vi "SA40144E.20210819 1D + 2D vacuum.vi"() -> ()   [LabVIEW 2020]
uses:
  <vilib>/Analysis/baseanly.llb/Mean (DBL).vi
  <userlib>/_OpenG.lib/file/file.llb/Build Path - Traditional__ogtk.vi
  <userlib>/LevyLab/LV to ITX/Data/Data.lvclass
  <userlib>/LevyLab/XY Utilities/xy_utilities.lvlib
  <vilib>/Analysis/NI_AALBase.lvlib
panel:
  in  "Tab Control":enum32{"Page 1", "Page 2"}(tab)
  out "Temp vs t":T1(graph)
  out "G4T vs t  2D":T1(graph)
  out "G2T vs t 2D":T1(graph)
  out "G4T vs t":T1(graph)
  out "G2T vs t":T1(graph)
  out "Lifespan vs Temp (hrs)":cluster{i32[], dbl[]}[](graph)
  out "Linear Fit 2T":T1(graph)
  out "Linear Fit 4T":T1(graph)
  out "Linear Fit 2D 4T":T1(graph)
  out "Arrhenius 0 V before T change":T1(graph)
  out "Arrhenius -50 V inc":T1(graph)
  out "Arrhenius -100 V":T1(graph)
  out "Arrhenius -50 V dec":T1(graph)
  out "Arrhenius middle 0":T1(graph)
  out "Arrhenius 50 V dec":T1(graph)
  out "Arrhenius 100 V":T1(graph)
  out "Arrhenius  50 V inc":T1(graph)
  out "Arrhenius - 0 V after T change":T1(graph)
  in  "Temps to keep (Lifespan)":i32=26
  in  "Source Voltage":dbl=0.01
  in  "Init Temp":i32=275
  in  "Temp Step":i32=5
  in  "Final Temp":i32=315
  in  "Data Folder":path=path "G:/My Drive/ansom/Data/PPMS 2/SA40144E.20210819/00 - test"
  in  "Trimming":i32=400
  in  "Update":bool
  in  "OK":bool
  out "error out":errorcluster
  in  "error in (no error)":errorcluster
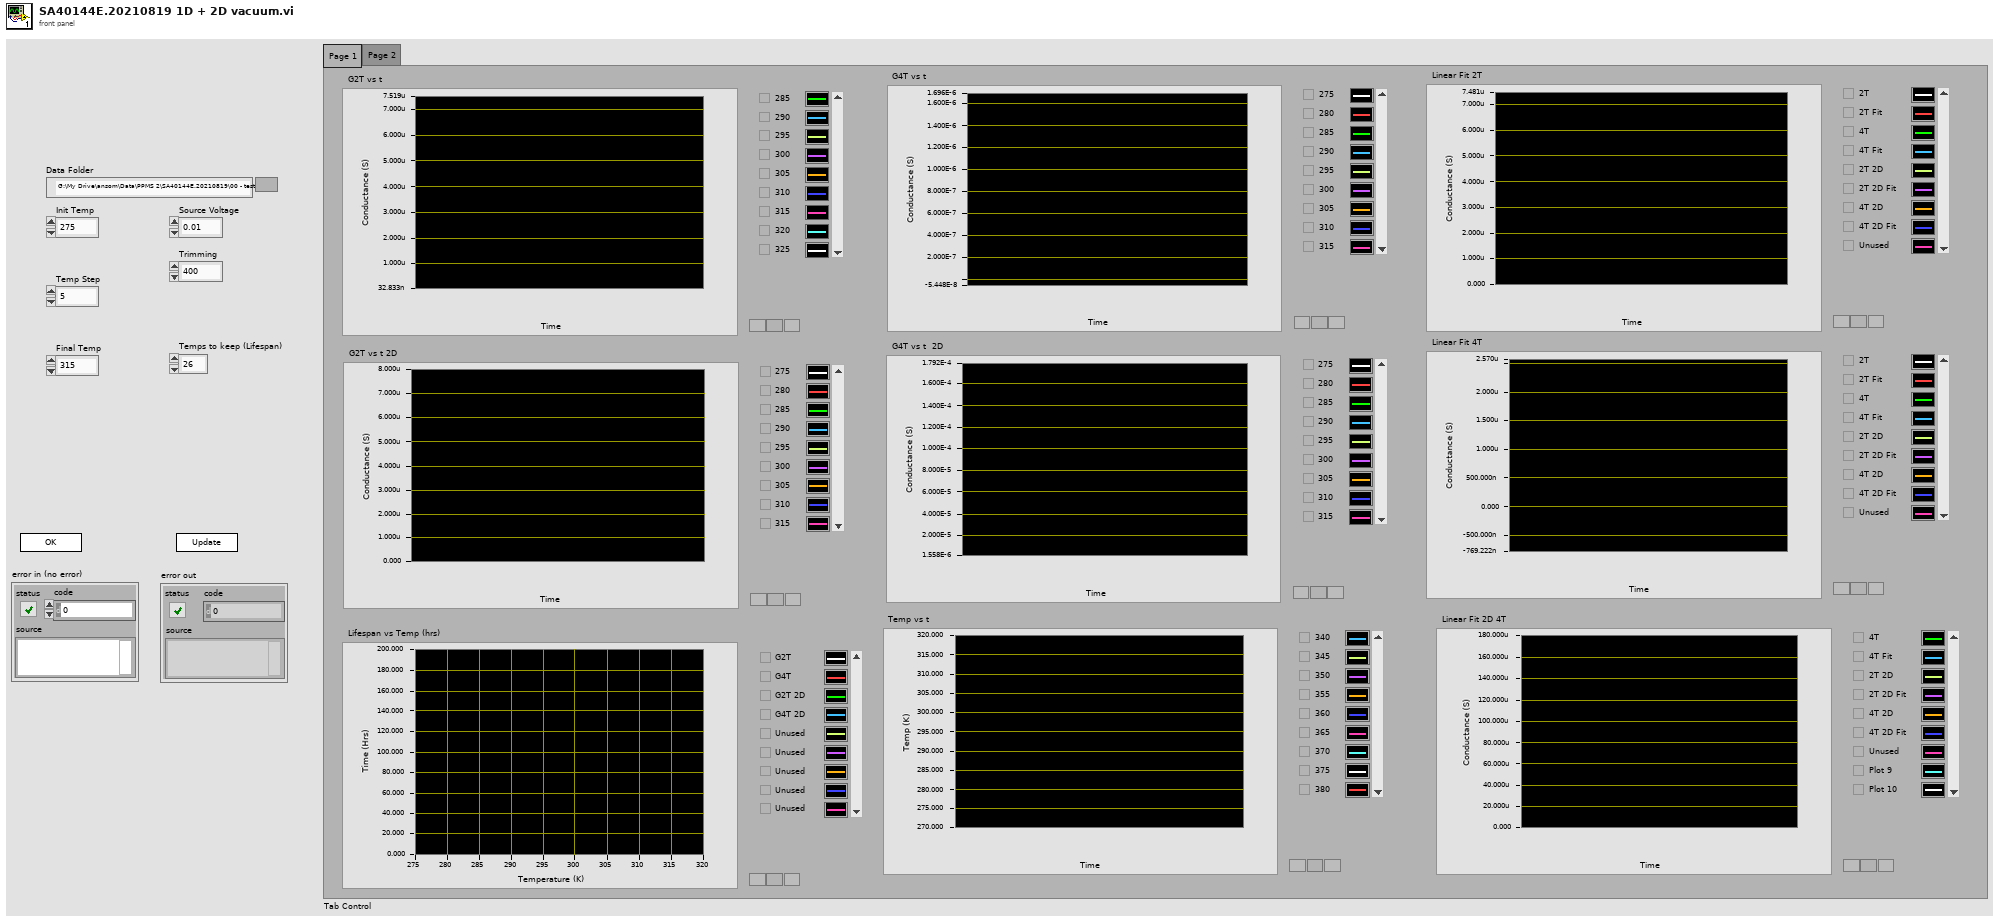
[diagram p1: front panel]
types:
  T1 = cluster{"Data":dbl[], "Best Exponential Fit":dbl[]}[]
  T2 = enum32{"Invalid", "Standard", "Closed", "Hidden", "Minimized", "Maximized"}
  T3 = enum32{"invalid app kind", "Development System", "Run Time System", "Student Edition", "Embedded LabVIEW", "Evaluation", "Custom"}
  T4 = cluster{"Core":cluster{"Current VI Reference":refnum<vi>, "Close Panel on Exit?":bool}, "G2T 1D":cluster{dbl[], dbl[]}[], "G4T 1D":cluster{dbl[], dbl[]}[], "G2T 2D":cluster{dbl[], dbl[]}[], "G4T 2D":cluster{dbl[], dbl[]}[], "Temp":cluster{dbl[], dbl[]}[], "Source Voltage":dbl, "Final Temp":i32, "Init Temp":i32, "Temp Step":i32, "Data Folder":path, "Trimming":i32}
  T5 = cluster{"Current VI Reference":refnum<vi>, "Close Panel on Exit?":bool}
  T6 = typedef "Data.lvclass/Dictionary--cluster.ctl" = cluster{"key":string, "value":variant}
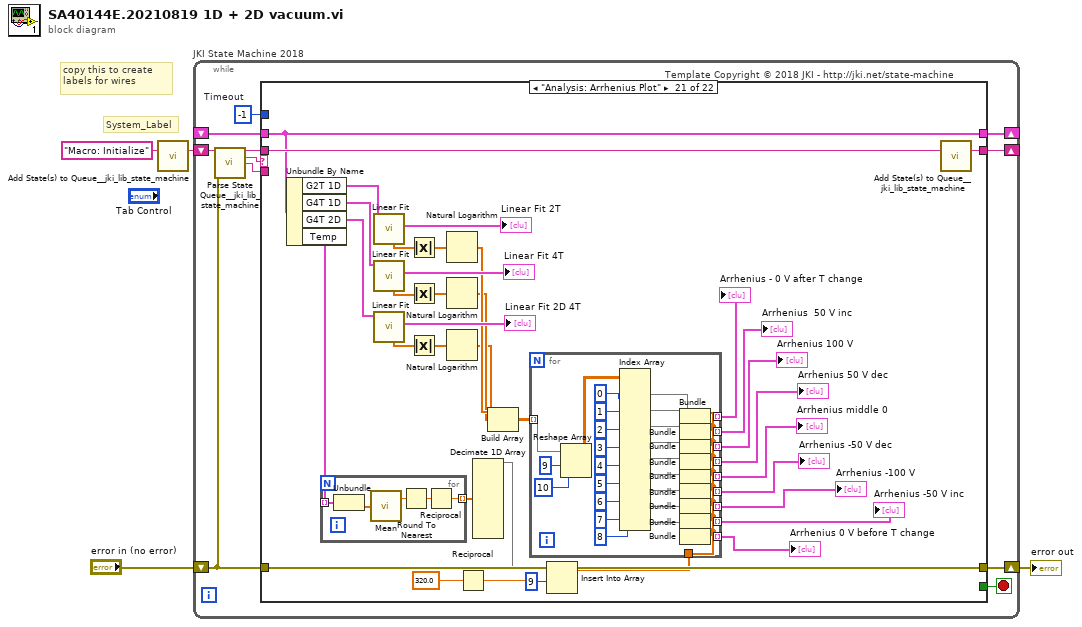
[diagram p0: block diagram]
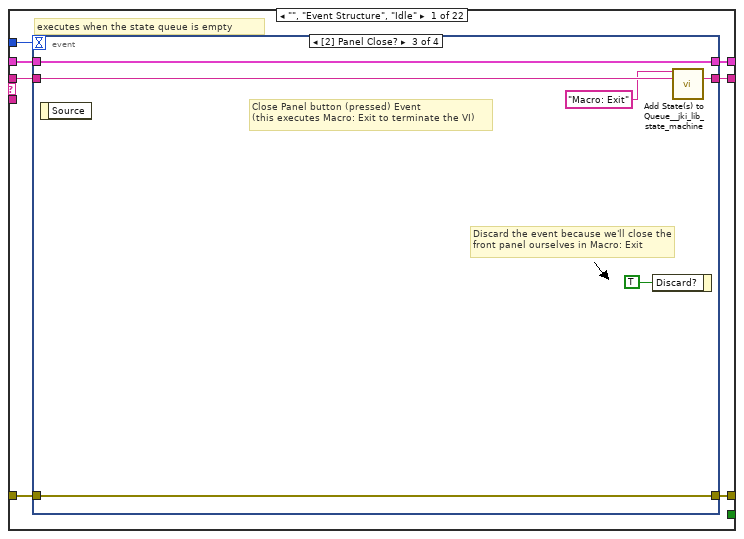
[diagram p2: hidden frame]
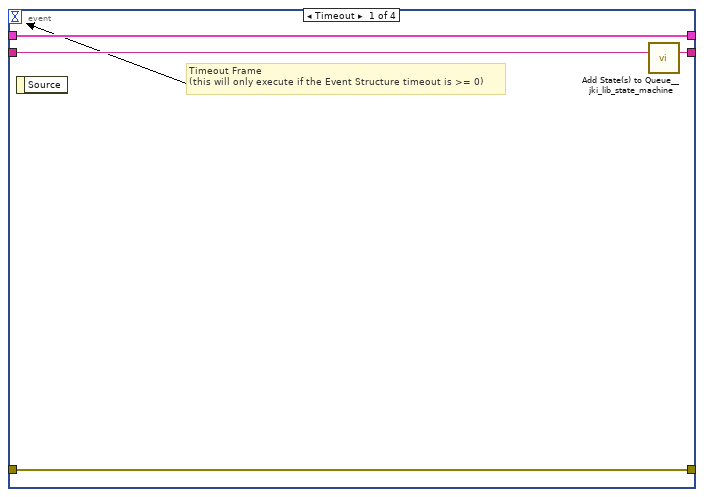
[diagram p3: hidden frame]
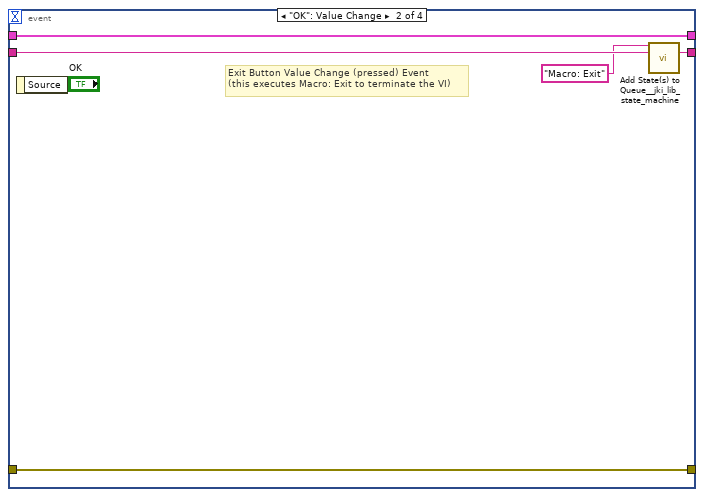
[diagram p4: hidden frame]
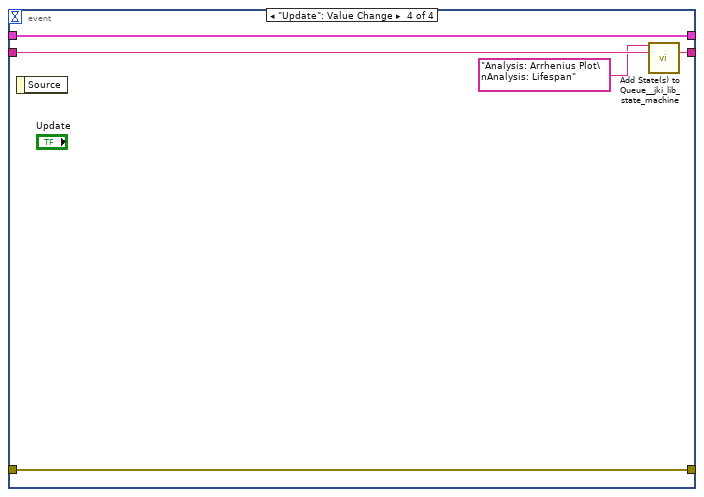
[diagram p5: hidden frame]
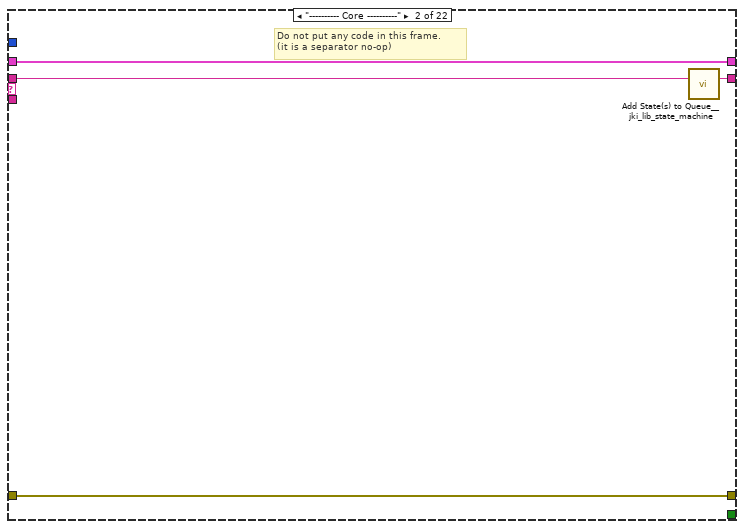
[diagram p6: hidden frame]
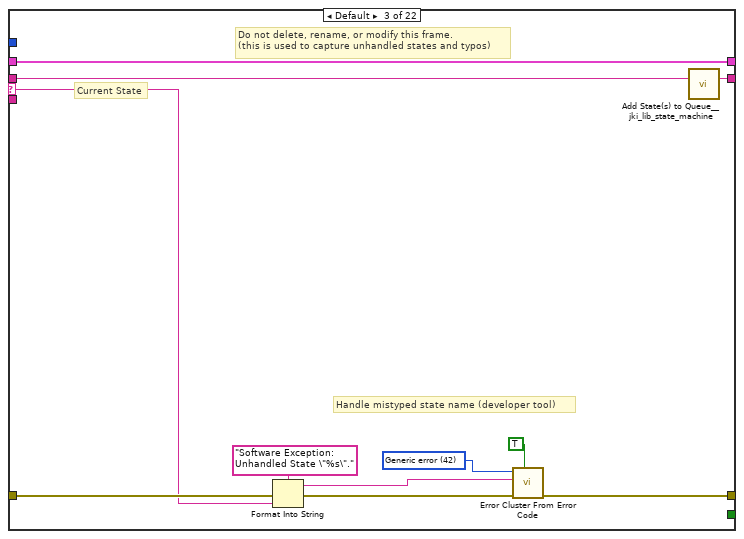
[diagram p7: hidden frame]
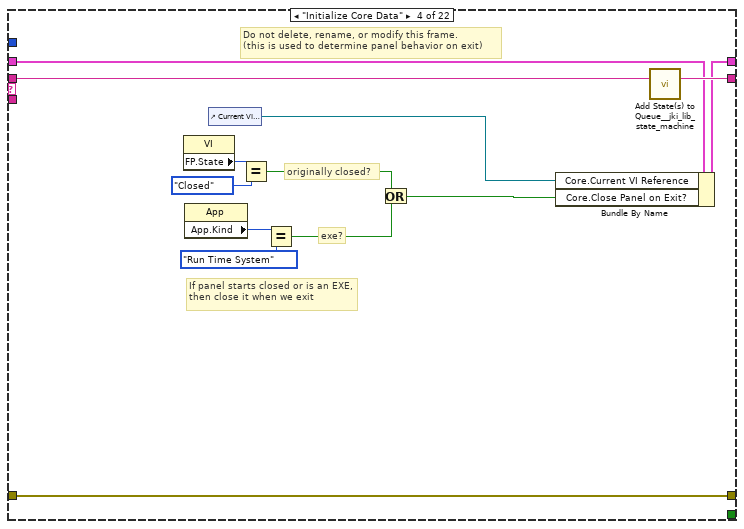
[diagram p8: hidden frame]
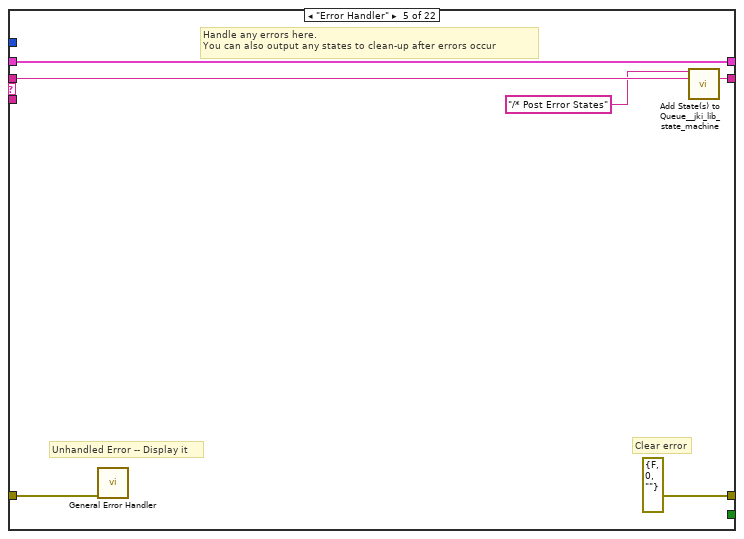
[diagram p9: hidden frame]
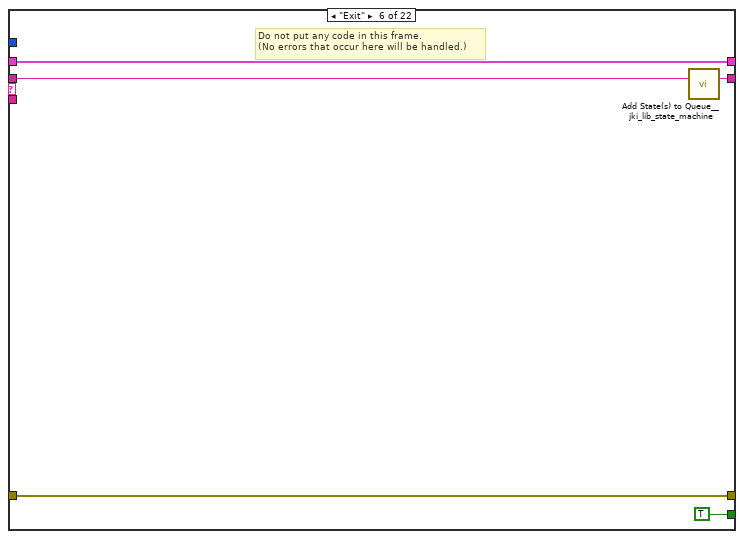
[diagram p10: hidden frame]
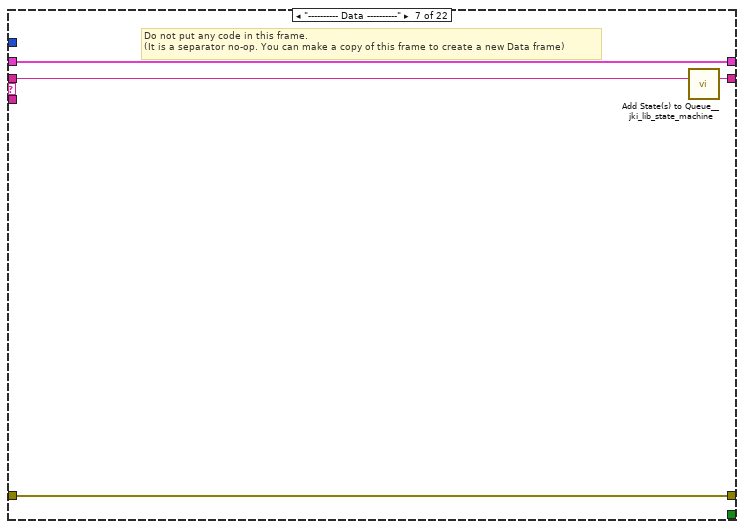
[diagram p11: hidden frame]
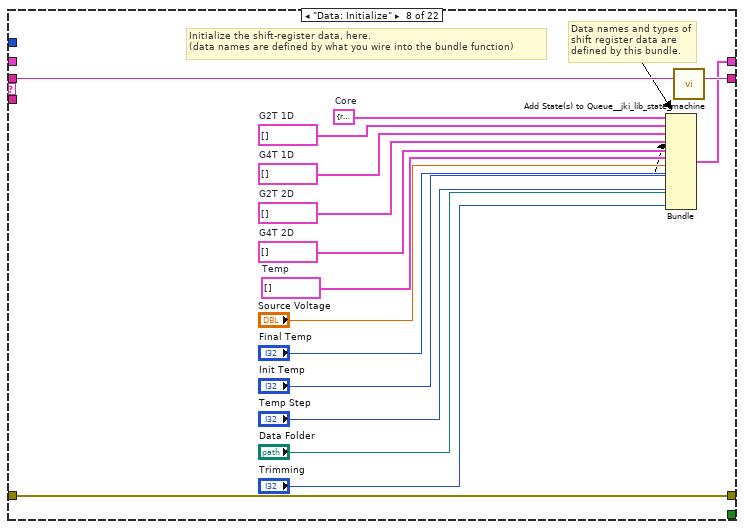
[diagram p12: hidden frame]
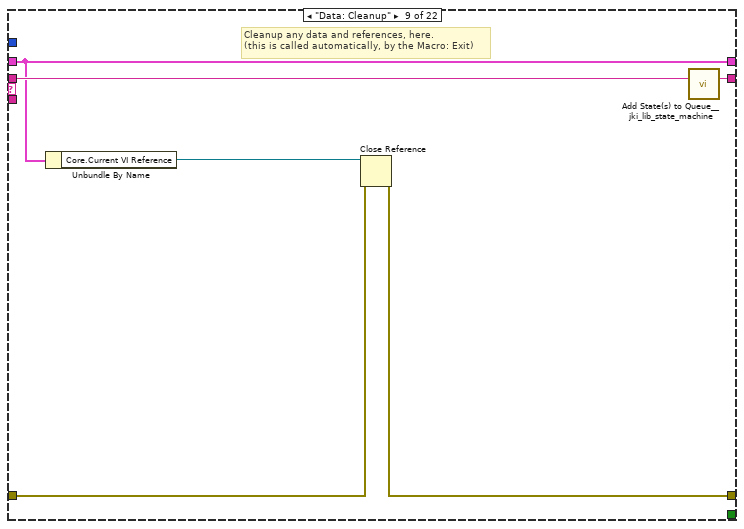
[diagram p13: hidden frame]
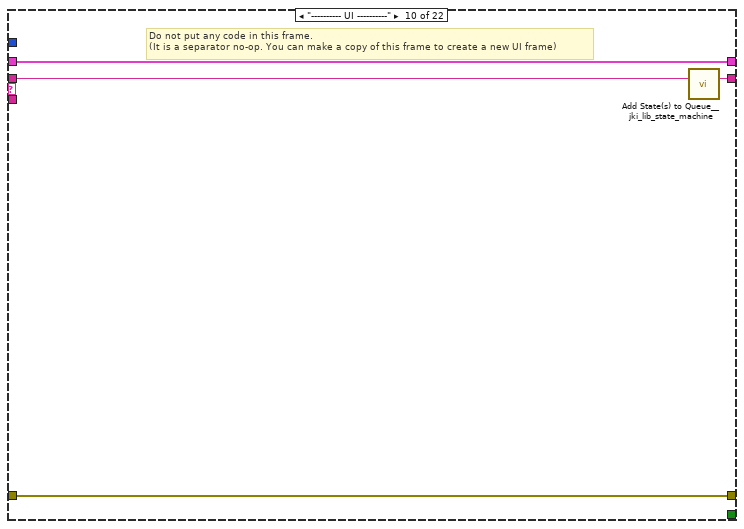
[diagram p14: hidden frame]
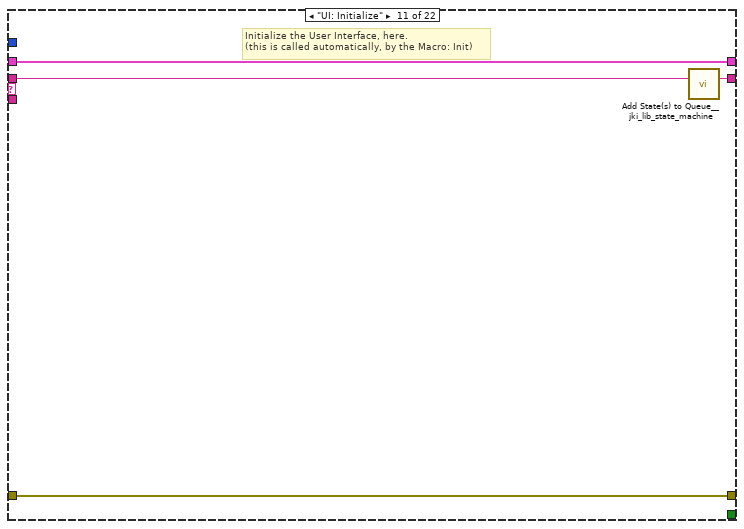
[diagram p15: hidden frame]
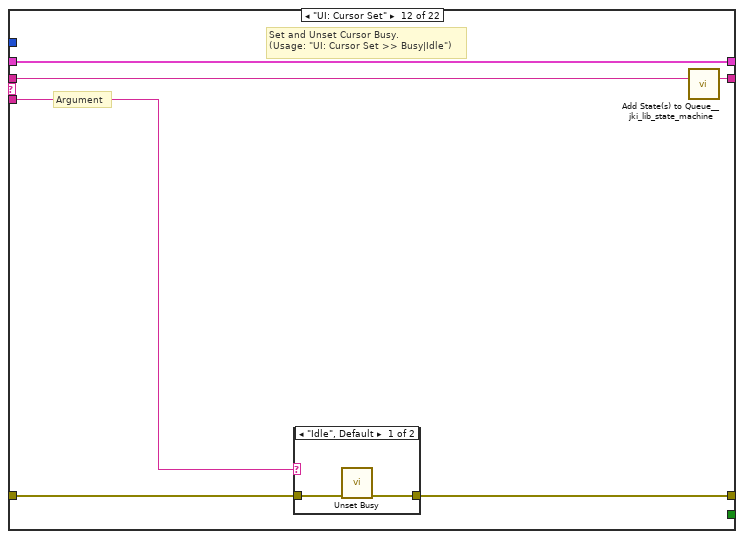
[diagram p16: hidden frame]
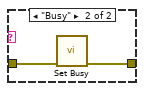
[diagram p17: hidden frame]
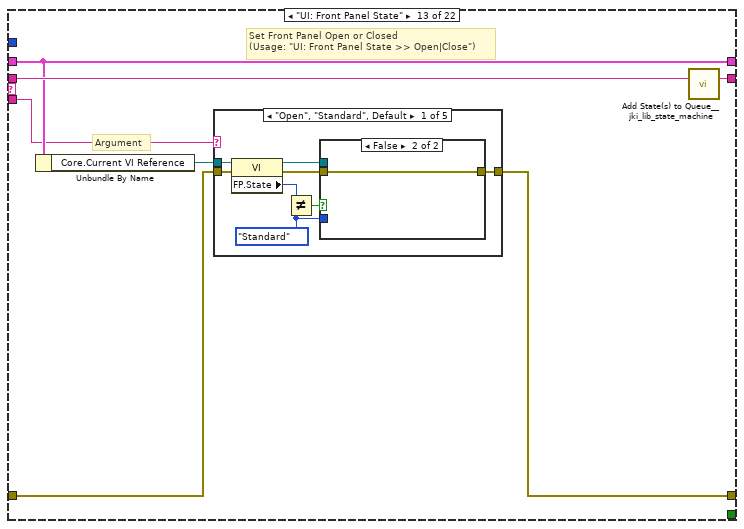
[diagram p18: hidden frame]
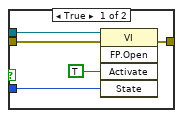
[diagram p19: hidden frame]
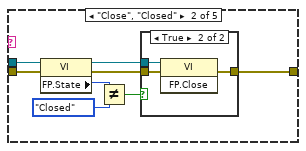
[diagram p20: hidden frame]
diagram:
  # "copy this to create labels for wires"
  # "System_Label"
  n1 = call <vilib>:"Add State(s) to Queue__jki_lib_state_machine.vi"("State(s) in (\"\")"="Macro: Initialize") -> ("States Out"=w4:string)  [unwired: 14 in]
  n2 = while "JKI State Machine 2018" {
    shift-right: [w8] -> _
    shift-left: _ -> [w7]
    shift-right: [w11] -> w1
    shift-left: "error in (no error)" -> [w5]
    shift-right: [w10] -> _
    shift-left: w4 -> [w12]
    stop <- w9 stop-if-true
    w6 = -1  # Timeout
    # "Template Copyright © 2018 JKI - http://jki.net/state-machine"
    n3 = call <vilib>:"Parse State Queue__jki_lib_state_machine.vi"("State Queue"=w12, "Error In (no error)"=w5) -> ("Remaining States"=w14:string, "Current State"=w15:string, "Arguments"=w13:string)  [unwired: 11 in]
    n4 = case shown="\"Analysis: Arrhenius Plot\"" w15 {
      selector: w15 -> [_ _ w47 _ _ _ _ _ _ _ _ _ _ _ _ _ _ _ _ _ _ _]
      tunnel: w14 -> [w22 w46 w51 w70 w76 w81 w85 w101 w107 w111 w115 w121 w132 w201 w206 w216 w220 w234 w274 w306 w342 w430]
      tunnel: w13 -> [_ _ _ _ _ _ _ _ _ _ _ w116 w126 _ _ _ _ _ _ _ _ _]
      tunnel: w7 -> [w20 w43 w49 w63 w73 w79 w82 _ w102 w108 w113 w119 w128 w198 w203 w213 w217 w230 w269 w303 w339 w410]
      tunnel: [w19 w44 w53 w67 errorcluster {"status"=FALSE, "code"=0, "source"=""} ("error out") w78 w83 w98 w103 w109 w112 w117 w129 w199 w204 w214 w218 w232 w272 w304 w340 w428] -> w11
      tunnel: w5 -> [w18 w44 w52 w67 w72 w78 w83 w98 w104 w109 w112 w118 w130 w199 w204 w214 w218 w232 w272 w304 w340 w428]
      tunnel: [w21 w45 w50 w69 w75 w80 w84 w100 w106 w110 w114 w120 w131 w200 w205 w215 w219 w233 w273 w305 w341 w429] -> w10
      tunnel: [_ _ _ _ _ TRUE _ _ _ _ _ _ _ _ _ _ _ _ _ _ _ _] -> w9
      tunnel: [w17 w43 w49 w68 w73 w79 w82 w99 w102 w108 w113 w119 w128 w198 w203 w213 w217 w231 w270 w303 w339 w410] -> w8
      tunnel: w6 -> [w16 _ _ _ _ _ _ _ _ _ _ _ _ _ _ _ _ _ _ _ _ _]
      frame "", "Event Structure", "Idle" {
        # "executes when the state queue is empty"
        n5 = event shown="[2] Panel Close?" {
          selector: _ -> [_ _ _ _]
          dyn-events: _ -> [_ _ _ _]
          timeout: w16 -> [_ _ _ _]
          tunnel: w22 -> [w26 w31 w37 w41]
          tunnel: [w25 w30 w36 w40] -> w21
          tunnel: w20 -> [w23 w28 w34 w42]
          tunnel: [w24 w29 w35 w38] -> w19
          tunnel: w18 -> [w24 w29 w35 w38]
          tunnel: [w23 w28 w34 w42] -> w17
          event Timeout {
            # "Timeout Frame\n(this will only execute if the Event Structure timeout is >= 0)"
            n6 = event-data() -> ()  [unwired: 1 in, 1 out]
            n7 = call <vilib>:"Add State(s) to Queue__jki_lib_state_machine.vi"("State(s) in (\"\")"=w26) -> ("States Out"=w25:string)  [unwired: 14 in]
          }
          event "OK": Value Change {
            # "Exit Button Value Change (pressed) Event\n(this executes Macro: Exit to terminate the VI)"
            n8 = event-data() -> ()  [unwired: 1 in, 1 out]
            n9 = call <vilib>:"Add State(s) to Queue__jki_lib_state_machine.vi"("State(s) in Front (\"\")"="Macro: Exit", "State(s) in (\"\")"=w31) -> ("States Out"=w30:string)  [unwired: 13 in]
          }
          event Panel Close? {
            # "Discard the event because we'll close the front panel ourselves in Macro: Exit"
            # "Close Panel button (pressed) Event\n(this executes Macro: Exit to terminate the VI)"
            n10 = event-data() -> ()  [unwired: 1 in, 1 out]
            n11 = event-data("Discard?"=TRUE) -> ()  [unwired: 1 in, 1 out]
            n12 = call <vilib>:"Add State(s) to Queue__jki_lib_state_machine.vi"("State(s) in Front (\"\")"="Macro: Exit", "State(s) in (\"\")"=w37) -> ("States Out"=w36:string)  [unwired: 13 in]
          }
          event "Update": Value Change {
            n13 = event-data() -> ()  [unwired: 1 in, 1 out]
            n14 = call <vilib>:"Add State(s) to Queue__jki_lib_state_machine.vi"("State(s) in Front (\"\")"="Analysis: Arrhenius Plot\nAnalysis: Lifespan" ("State(s) in Front (\"\")"), "State(s) in (\"\")"=w41) -> ("States Out"=w40:string)  [unwired: 13 in]
          }
        }
      }
      frame "---------- Core ----------" {
        # "Do not put any code in this frame.\n(it is a separator no-op)"
        n15 = call <vilib>:"Add State(s) to Queue__jki_lib_state_machine.vi"("State(s) in (\"\")"=w46) -> ("States Out"=w45:string)  [unwired: 14 in]
      }
      frame Default {
        w56 = 42 items=["No error", "Argument error", "Memory is full", "Out of zone", "End of file", "File already open", "Generic file I/O error", "File not found", "File permission error", "Disk is full", "Duplicate path", "Too many files open", "System feature not enabled", "Resource file not found", "Cannot add resource", "Resource not found", "Image not found", "Image memory error", "Pen does not exist", "Config type invalid", "Config token not found", "Config parse error", "Config memory error", "Bad external code format", "Bad external code offset", "External code not present", "Null window", "Destroy window error", "Null menu", "Print aborted", "Bad print record", "Print driver error", "Windows error during printing", "Memory error during printing", "Print dialog error", "Generic print error", "Invalid device refnum", "Device not found", "Device parameter error", "Device unit error", "Cannot open device", "Device call aborted", "Generic error", "Cancelled by user", "Object ID too low", "Object ID too high", "Object not in heap", "Unknown heap", "Unknown object (invalid DefProc)", "Unknown object (DefProc not in table)", "Message out of range", "Invalid (null) method", "Unknown message", "Manager call not supported", "Bad address", "Network operation in progress", "Network operation timed out", "Connection is busy", "Network attribute not supported", "Network error", "Address in use", "System out of memory", "Connection aborted", "Connection refused", "Not connected", "Already connected", "Connection closed", "Initialization error (interapplication manager)", "Bad occurrence", "Wait on unbound occurrence handler", "Occurrence queue overflow", "Datalog type conflict", "Unused", "Unrecognized type (interapplication manager)", "Memory corrupt", "Failed to make temporary DLL", "Old CIN version", "Drag socket not found", "Failed to load drop-object", "Failed to register OLE object", "Failed to release OLE object", "Format specifier type mismatch", "Unknown format specifier", "Too few format specifiers", "Too many format specifiers", "Scan failed", "Newer CIN version", "Error converting to variant", "Runtime menu error", "Password tampered", "Variant attribute not found", "Incompatible variant data type", "Event data is not available", "Event Store is not present", "Occurrence is not found", "Event Queue is not created", "Event info is not available", "Refnum passed is NULL", "Error retrieving Class GUID", "Error retrieving CoClass GUID", "Error retrieving TypeLib GUID.", "Bad built application magic bytes.", "Specific driver is different from the specific driver associated with the Logical Name.", "There is no session opened to the class driver.", "Max Error", "MAX - Error with config objects", "MAX - Error loading configuration", "MAX - Group not supported"]
        # "Current State"
        # "Do not delete, rename, or modify this frame.\n(this is used to capture unhandled states and typos)"
        # "Handle mistyped state name (developer tool)"
        n16 = Format Into String(format string="Software Exception: Unhandled State \"%s\"." ("message"), error in=w52, w47) -> (resulting string=w55:string, error out=w54:errorcluster)  [unwired: 1 in]
        n17 = call <vilib>:"Error Cluster From Error Code.vi"("show call chain? (False)"=TRUE, "error in (no error)"=w54, "error message (\"\")"=w55, "error code (0)"=w56) -> ("error out"=w53:errorcluster)  [unwired: 5 in]
        n18 = call <vilib>:"Add State(s) to Queue__jki_lib_state_machine.vi"("State(s) in (\"\")"=w51) -> ("States Out"=w50:string)  [unwired: 14 in]
      }
      frame "Initialize Core Data" {
        # "Do not delete, rename, or modify this frame.\n(this is used to determine panel behavior on exit)"
        # "originally closed?"
        # "exe?"
        # "If panel starts closed or is an EXE, then close it when we exit"
        n19 = property class="VI"() -> ("FP.State"=w60:T2)  [unwired: 2 in, 2 out]
        n20 = property class="App"() -> ("App.Kind"=w66:T3)  [unwired: 2 in, 2 out]
        n21 = control-ref of="Current VI Reference"() -> (w61:refnum<vi>)
        n22 = Equal?(x=w60, y=T2."Closed" ("Front Panel Window:State")) -> (x = y?=w58:bool)
        n23 = Equal?(x=w66, y=T3."Run Time System" ("Application:Kind")) -> (x = y?=w64:bool)
        n24 = Or(x=w58, y=w64) -> (x .or. y?=w62:bool)
        n25 = Bundle By Name(cluster=w63, "Core.Current VI Reference"=w61, "Core.Close Panel on Exit?"=w62) -> (w68:T4)
        n26 = call <vilib>:"Add State(s) to Queue__jki_lib_state_machine.vi"("State(s) in (\"\")"=w70) -> ("States Out"=w69:string)  [unwired: 14 in]
      }
      frame "Error Handler" {
        # "Unhandled Error -- Display it"
        # "Handle any errors here.\nYou can also output any states to clean-up after errors occur"
        # "Clear error"
        n27 = call <vilib>:"General Error Handler.vi"("error in (no error)"=w72) -> ()  [unwired: 10 in, 5 out]
        n28 = call <vilib>:"Add State(s) to Queue__jki_lib_state_machine.vi"("State(s) in Front (\"\")"="/* Post Error States", "State(s) in (\"\")"=w76) -> ("States Out"=w75:string)  [unwired: 13 in]
      }
      frame "Exit" {
        # "Do not put any code in this frame.\n(No errors that occur here will be handled.)"
        n29 = call <vilib>:"Add State(s) to Queue__jki_lib_state_machine.vi"("State(s) in (\"\")"=w81) -> ("States Out"=w80:string)  [unwired: 14 in]
      }
      frame "---------- Data ----------" {
        # "Do not put any code in this frame.\n(It is a separator no-op. You can make a copy of this frame to create a new Data frame)"
        n30 = call <vilib>:"Add State(s) to Queue__jki_lib_state_machine.vi"("State(s) in (\"\")"=w85) -> ("States Out"=w84:string)  [unwired: 14 in]
      }
      frame "Data: Initialize" {
        w86 = cluster{dbl[], dbl[]}[] []  # Temp
        w95 = cluster{dbl[], dbl[]}[] []  # G4T 2D
        w94 = cluster{dbl[], dbl[]}[] []  # G2T 2D
        w93 = cluster{dbl[], dbl[]}[] []  # G4T 1D
        w92 = cluster{dbl[], dbl[]}[] []  # G2T 1D
        w97 = T5 {"Current VI Reference"=refnum, "Close Panel on Exit?"=FALSE}  # Core
        # "Data names and types of shift register data are defined by this bundle."
        # "Initialize the shift-register data, here.\n(data names are defined by what you wire into the bundle function)"
        n31 = Bundle("Core"=w97, "G2T 1D"=w92, "G4T 1D"=w93, "G2T 2D"=w94, "G4T 2D"=w95, "Temp"=w86, "Source Voltage"="Source Voltage", "Final Temp"="Final Temp", "Init Temp"="Init Temp", "Temp Step"="Temp Step", "Data Folder"="Data Folder", "Trimming"="Trimming") -> (w99:T4)  [unwired: 1 in]
        n32 = call <vilib>:"Add State(s) to Queue__jki_lib_state_machine.vi"("State(s) in (\"\")"=w101) -> ("States Out"=w100:string)  [unwired: 14 in]
      }
      frame "Data: Cleanup" {
        # "Cleanup any data and references, here.\n(this is called automatically, by the Macro: Exit)"
        n33 = Unbundle By Name(w102) -> ("Core.Current VI Reference"=w105:refnum<vi>)
        n34 = Close Reference(reference=w105, error in (no error)=w104) -> (error out=w103:errorcluster)
        n35 = call <vilib>:"Add State(s) to Queue__jki_lib_state_machine.vi"("State(s) in (\"\")"=w107) -> ("States Out"=w106:string)  [unwired: 14 in]
      }
      frame "---------- UI ----------" {
        # "Do not put any code in this frame.\n(It is a separator no-op. You can make a copy of this frame to create a new UI frame)"
        n36 = call <vilib>:"Add State(s) to Queue__jki_lib_state_machine.vi"("State(s) in (\"\")"=w111) -> ("States Out"=w110:string)  [unwired: 14 in]
      }
      frame "UI: Initialize" {
        # "Initialize the User Interface, here.\n(this is called automatically, by the Macro: Init)"
        n37 = call <vilib>:"Add State(s) to Queue__jki_lib_state_machine.vi"("State(s) in (\"\")"=w115) -> ("States Out"=w114:string)  [unwired: 14 in]
      }
      frame "UI: Cursor Set" {
        # "Argument"
        # "Set and Unset Cursor Busy.\n(Usage: \"UI: Cursor Set >> Busy|Idle\")"
        n38 = case shown="\"Idle\", Default" w116 {
          tunnel: w118 -> [w123 w125]
          tunnel: [w122 w124] -> w117
          frame "Idle", Default {
            n39 = call <vilib>:"Unset Busy.vi"("error in (no error)"=w123) -> ("error out"=w122:errorcluster)  [unwired: 10 in]
          }
          frame "Busy" {
            n40 = call <vilib>:"Set Busy.vi"("error in (no error)"=w125) -> ("error out"=w124:errorcluster)  [unwired: 9 in, 1 out]
          }
        }
        n41 = call <vilib>:"Add State(s) to Queue__jki_lib_state_machine.vi"("State(s) in (\"\")"=w121) -> ("States Out"=w120:string)  [unwired: 14 in]
      }
      frame "UI: Front Panel State" {
        # "Argument"
        # "Set Front Panel Open or Closed\n(Usage: \"UI: Front Panel State >> Open|Close\")"
        n42 = Unbundle By Name(w128) -> ("Core.Current VI Reference"=w127:refnum<vi>)
        n43 = case shown="\"Open\", \"Standard\", Default" w126 {
          tunnel: w130 -> [w138 w153 w164 w177 w190]
          tunnel: [w140 w154 w166 w179 w192] -> w129
          tunnel: w127 -> [w139 w151 w165 w178 w191]
          frame "Open", "Standard", Default {
            w133 = T2."Standard" ("State")
            n44 = property class="VI"(reference=w139, error in=w138) -> (reference out=w136:refnum<vi>, error out=w137:errorcluster, "FP.State"=w135:T2)
            n45 = Not Equal?(x=w135, y=w133) -> (x != y?=w134:bool)
            n46 = case shown="False" w134 {
              tunnel: [w144 w146] -> w140
              tunnel: w137 -> [w143 w146]
              tunnel: w136 -> [w142 _]
              tunnel: w133 -> [w141 _]
              frame True {
                n47 = invoke class="VI" method="FP.Open"(reference=w142, error in=w143, "Activate"=TRUE, "State"=w141) -> (error out=w144:errorcluster)  [unwired: 1 in, 4 out]
              }
              frame False {
              }
            }
          }
          frame "Close", "Closed" {
            n48 = property class="VI"(reference=w151, error in=w153) -> (reference out=w150:refnum<vi>, error out=w152:errorcluster, "FP.State"=w148:T2)
            n49 = Not Equal?(x=w148, y=T2."Closed" ("Front Panel Window:State")) -> (x != y?=w147:bool)
            n50 = case shown="True" w147 {
              tunnel: [w155 w158] -> w154
              tunnel: w152 -> [w155 w157]
              tunnel: w150 -> [_ w156]
              frame False {
              }
              frame True {
                n51 = invoke class="VI" method="FP.Close"(reference=w156, error in=w157) -> (error out=w158:errorcluster)  [unwired: 1 in, 2 out]
              }
            }
          }
          frame "Hidden", "Hide" {
            w159 = T2."Hidden" ("State")
            n52 = property class="VI"(reference=w165, error in=w164) -> (reference out=w162:refnum<vi>, error out=w163:errorcluster, "FP.State"=w161:T2)
            n53 = Not Equal?(x=w161, y=w159) -> (x != y?=w160:bool)
            n54 = case shown="True" w160 {
              tunnel: [w170 w171] -> w166
              tunnel: w163 -> [w169 w171]
              tunnel: w162 -> [w168 _]
              tunnel: w159 -> [w167 _]
              frame True {
                n55 = invoke class="VI" method="FP.Open"(reference=w168, error in=w169, "State"=w167) -> (error out=w170:errorcluster)  [unwired: 2 in, 4 out]
              }
              frame False {
              }
            }
          }
          frame "Minimize", "Minimized" {
            w172 = T2."Minimized" ("State")
            n56 = property class="VI"(reference=w178, error in=w177) -> (reference out=w175:refnum<vi>, error out=w176:errorcluster, "FP.State"=w174:T2)
            n57 = Not Equal?(x=w174, y=w172) -> (x != y?=w173:bool)
            n58 = case shown="True" w173 {
              tunnel: [w183 w184] -> w179
              tunnel: w176 -> [w182 w184]
              tunnel: w175 -> [w181 _]
              tunnel: w172 -> [w180 _]
              frame True {
                n59 = invoke class="VI" method="FP.Open"(reference=w181, error in=w182, "State"=w180) -> (error out=w183:errorcluster)  [unwired: 2 in, 4 out]
              }
              frame False {
              }
            }
          }
          frame "Maximize", "Maximized" {
            w185 = T2."Maximized" ("State")
            n60 = property class="VI"(reference=w191, error in=w190) -> (reference out=w188:refnum<vi>, error out=w189:errorcluster, "FP.State"=w187:T2)
            n61 = Not Equal?(x=w187, y=w185) -> (x != y?=w186:bool)
            n62 = case shown="True" w186 {
              tunnel: [w196 w197] -> w192
              tunnel: w189 -> [w195 w197]
              tunnel: w188 -> [w194 _]
              tunnel: w185 -> [w193 _]
              frame True {
                n63 = invoke class="VI" method="FP.Open"(reference=w194, error in=w195, "State"=w193) -> (error out=w196:errorcluster)  [unwired: 2 in, 4 out]
              }
              frame False {
              }
            }
          }
        }
        n64 = call <vilib>:"Add State(s) to Queue__jki_lib_state_machine.vi"("State(s) in (\"\")"=w132) -> ("States Out"=w131:string)  [unwired: 14 in]
      }
      frame "---------- Macro ----------" {
        # "Do not put any code in this frame.\n(It is a separator no-op. You can make a copy of this frame to create a new Macro frame)"
        n65 = call <vilib>:"Add State(s) to Queue__jki_lib_state_machine.vi"("State(s) in (\"\")"=w201) -> ("States Out"=w200:string)  [unwired: 14 in]
      }
      frame "Macro: Initialize" {
        # "Initialization Macro\n(This is called once, when the VI starts)"
        n66 = call <vilib>:"Add State(s) to Queue__jki_lib_state_machine.vi"("State(s) in Front (\"\")"="Data: Initialize\nInitialize Core Data\nUI: Initialize\nUI: Front Panel State >> Open\nAnalysis: Load 1D\nAnalysis: Load 2D\nAnalysis: Plot G vs t\nAnalysis: Arrhenius Plot\n# Analysis: Lifespan", "State(s) in (\"\")"=w206) -> ("States Out"=w205:string)  [unwired: 13 in]
      }
      frame "Macro: Exit" {
        # "Exit Macro\n(This is called once, when the VI exits)"
        n67 = Unbundle By Name(w213) -> ("Core.Close Panel on Exit?"=w212:bool)
        n68 = Select(t="UI: Front Panel State >> Close", s=w212, f="") -> (s? t:f=w209:string)
        n69 = call <vilib>:"Add State(s) to Queue__jki_lib_state_machine.vi"("State(s) in (\"\")"=w209, "State(s) at Back (\"\")"="Data: Cleanup\nExit") -> ("States Out"=w207:string)  [unwired: 13 in]
        n70 = call <vilib>:"Add State(s) to Queue__jki_lib_state_machine.vi"("State(s) in Front (\"\")"=w207, "State(s) in (\"\")"=w216) -> ("States Out"=w215:string)  [unwired: 13 in]
      }
      frame "---------- Analysis ----------" {
        # "Template Separator\n(You can make a copy of, or modify, this frame)"
        n71 = call <vilib>:"Add State(s) to Queue__jki_lib_state_machine.vi"("State(s) in (\"\")"=w220) -> ("States Out"=w219:string)  [unwired: 14 in]
      }
      frame "Analysis: Load 1D" {
        # "G2T = X3/V_s\nG4T = X3/(X5-X4)"
        n72 = Unbundle By Name(w230) -> ("Source Voltage"=w229:dbl, "Trimming"=w225:i32, "Data Folder"=w226:path)
        n73 = List Folder(path=w226, pattern="*.dat") -> (path out=w224:path, filenames=w223:string[])  [unwired: 2 in, 2 out]
        n74 = for {
          tunnel: w229 -> [w240]
          tunnel: [w261] -> w228 mode=indexing
          tunnel: [w260] -> w222 mode=indexing
          tunnel: w225 -> [w246]
          tunnel: [w258] -> w227 mode=indexing
          tunnel: w224 -> [w245]
          tunnel: w223 -> [w244] mode=indexing
          n75 = call-poly <userlib>:"Build Path__ogtk.vi"("name or relative path"=w244, "base path"=w245) -> ("appended path"=w243:path)
          n76 = call <userlib>:"Data Read.vi"("path"=w243) -> ("Data (Dictionary)"=w257:T6[])  [unwired: 7 in, 3 out]
          n77 = call "Read Dictionary.vi"("Numeric"=0, "Dictionary In"=w257) -> ("data"=w253:dbl[])
          n78 = call "Read Dictionary.vi"("Numeric"=5, "Dictionary In"=w257) -> ("data"=w247:dbl[])
          n79 = call "Read Dictionary.vi"("Numeric"=7 ("index"), "Dictionary In"=w257) -> ("data"=w248:dbl[])
          n80 = call "Read Dictionary.vi"("Numeric"=6, "Dictionary In"=w257) -> ("data"=w252:dbl[])
          n81 = call "Read Dictionary.vi"("Numeric"=1, "Dictionary In"=w257) -> ("data"=w251:dbl[])
          n82 = Array Subset(array=w253, index=w246) -> (w242:dbl[])  [unwired: 1 in]
          n83 = Array Subset(array=w247, index=w246) -> (w237:dbl[])  [unwired: 1 in]
          n84 = Array Subset(array=w248, index=w246) -> (w239:dbl[])  [unwired: 1 in]
          n85 = Array Subset(array=w252, index=w246) -> (w238:dbl[])  [unwired: 1 in]
          n86 = Subtract(x=w239, y=w238) -> (x-y=w236:dbl[])
          n87 = Divide(x=w237, y=w240) -> (x/y=w241:dbl[])
          n88 = Divide(x=w237, y=w236) -> (x/y=w235:dbl[])
          n89 = Array Subset(array=w251) -> (w259:dbl[])  [unwired: 2 in]
          n90 = Bundle(w242, w241) -> (w261:cluster{dbl[], dbl[]})  [unwired: 1 in]
          n91 = Bundle(w242, w259) -> (w258:cluster{dbl[], dbl[]})  [unwired: 1 in]
          n92 = Bundle(w242, w235) -> (w260:cluster{dbl[], dbl[]})  [unwired: 1 in]
        }
        n93 = call <vilib>:"Add State(s) to Queue__jki_lib_state_machine.vi"("State(s) in (\"\")"=w234) -> ("States Out"=w233:string)  [unwired: 14 in]
        n94 = Bundle By Name(cluster=w230, "G2T 1D"=w228, "G4T 1D"=w222, "Temp"=w227) -> (w231:T4)
      }
      frame "Analysis: Load 2D" {
        # "G2T = X3/V_s\nG4T = X3/(X8-X1)"
        n95 = Unbundle By Name(w269) -> ("Source Voltage"=w271:dbl, "Trimming"=w268:i32, "Data Folder"=w267:path)
        n96 = List Folder(path=w267, pattern="*.dat") -> (path out=w266:path, filenames=w265:string[])  [unwired: 2 in, 2 out]
        n97 = for {
          tunnel: w271 -> [w279]
          tunnel: [w296] -> w264 mode=indexing
          tunnel: [w295] -> w263 mode=indexing
          tunnel: w268 -> [w294]
          tunnel: w266 -> [w283]
          tunnel: w265 -> [w282] mode=indexing
          n98 = call-poly <userlib>:"Build Path__ogtk.vi"("name or relative path"=w282, "base path"=w283) -> ("appended path"=w297:path)
          n99 = call <userlib>:"Data Read.vi"("path"=w297) -> ("Data (Dictionary)"=w292:T6[])  [unwired: 7 in, 3 out]
          n100 = call "Read Dictionary.vi"("Numeric"=0, "Dictionary In"=w292) -> ("data"=w291:dbl[])
          n101 = call "Read Dictionary.vi"("Numeric"=5, "Dictionary In"=w292) -> ("data"=w288:dbl[])
          n102 = call "Read Dictionary.vi"("Numeric"=3 ("index"), "Dictionary In"=w292) -> ("data"=w289:dbl[])
          n103 = call "Read Dictionary.vi"("Numeric"=4, "Dictionary In"=w292) -> ("data"=w290:dbl[])
          n104 = Array Subset(array=w291, index=w294) -> (w293:dbl[])  [unwired: 1 in]
          n105 = Array Subset(array=w288, index=w294) -> (w280:dbl[])  [unwired: 1 in]
          n106 = Array Subset(array=w289, index=w294) -> (w278:dbl[])  [unwired: 1 in]
          n107 = Array Subset(array=w290, index=w294) -> (w277:dbl[])  [unwired: 1 in]
          n108 = Subtract(x=w278, y=w277) -> (x-y=w281:dbl[])
          n109 = Divide(x=w280, y=w279) -> (x/y=w275:dbl[])
          n110 = Divide(x=w280, y=w281) -> (x/y=w276:dbl[])
          n111 = Bundle(w293, w275) -> (w296:cluster{dbl[], dbl[]})  [unwired: 1 in]
          n112 = Bundle(w293, w276) -> (w295:cluster{dbl[], dbl[]})  [unwired: 1 in]
        }
        n113 = call <vilib>:"Add State(s) to Queue__jki_lib_state_machine.vi"("State(s) in (\"\")"=w274) -> ("States Out"=w273:string)  [unwired: 14 in]
        n114 = Bundle By Name(cluster=w269, "G2T 2D"=w264, "G4T 2D"=w263) -> (w270:T4)
      }
      frame "Analysis: Plot G vs t" {
        n115 = Unbundle By Name(w303) -> ("G2T 1D"=→"G2T vs t":cluster{dbl[], dbl[]}[], "G4T 1D"=→"G4T vs t":cluster{dbl[], dbl[]}[], "G2T 2D"=→"G2T vs t 2D":cluster{dbl[], dbl[]}[], "G4T 2D"=→"G4T vs t  2D":cluster{dbl[], dbl[]}[], "Temp"=→"Temp vs t":cluster{dbl[], dbl[]}[])
        n116 = call <vilib>:"Add State(s) to Queue__jki_lib_state_machine.vi"("State(s) in (\"\")"=w306) -> ("States Out"=w305:string)  [unwired: 14 in]
      }
      frame "Analysis: Arrhenius Plot" {
        n117 = Unbundle By Name(w339) -> ("G2T 1D"=w336:cluster{dbl[], dbl[]}[], "G4T 1D"=w335:cluster{dbl[], dbl[]}[], "G4T 2D"=w338:cluster{dbl[], dbl[]}[], "Temp"=w329:cluster{dbl[], dbl[]}[])
        n118 = for {
          tunnel: w329 -> [w379] mode=indexing
          tunnel: [w377] -> w321 mode=indexing
          n119 = Unbundle(w379) -> (w376:dbl[])  [unwired: 1 out]
          n120 = call-poly <vilib>:"Mean.vi"("X"=w376) -> ("mean"=w375:dbl)  [unwired: 1 out]
          n121 = Round To Nearest(number=w375) -> (nearest integer value=w378:dbl)
          n122 = Reciprocal(x=w378) -> (1/x=w377:dbl)
        }
        n123 = call-poly <userlib>:"Linear Fit.vi"("XY-data"=w336) -> ("Best Fits"=→"Linear Fit 2T":cluster{"X-array":dbl[], "Y-array":dbl[]}[], "slopes"=w333:dbl[])  [unwired: 4 in, 5 out]
        n124 = call-poly <userlib>:"Linear Fit.vi"("XY-data"=w335) -> ("Best Fits"=→"Linear Fit 4T":cluster{"X-array":dbl[], "Y-array":dbl[]}[], "slopes"=w334:dbl[])  [unwired: 4 in, 5 out]
        n125 = call-poly <userlib>:"Linear Fit.vi"("XY-data"=w338) -> ("Best Fits"=→"Linear Fit 2D 4T":cluster{"X-array":dbl[], "Y-array":dbl[]}[], "slopes"=w337:dbl[])  [unwired: 4 in, 5 out]
        n126 = Absolute Value(x=w333) -> (abs(x)=w328:dbl[])
        n127 = Absolute Value(x=w334) -> (abs(x)=w327:dbl[])
        n128 = Absolute Value(x=w337) -> (abs(x)=w326:dbl[])
        n129 = Natural Logarithm(1:w328) -> (0:w324:dbl[])
        n130 = Natural Logarithm(1:w327) -> (0:w323:dbl[])
        n131 = Natural Logarithm(1:w326) -> (0:w322:dbl[])
        n132 = Reciprocal(x=320.0 ("new element/subarray")) -> (1/x=w317:dbl)
        n133 = Decimate 1D Array(w321) -> (w320:dbl[])  [unwired: 9 out]
        n134 = Build Array(w324, w323, w322) -> (w325:dbl[][])
        n135 = Insert Into Array(array=w320, index=9, new element=w317) -> (w316:dbl[])
        n136 = for {
          tunnel: w325 -> [w364] mode=indexing
          tunnel: w316 -> [w374]
          tunnel: [w373] -> w315 mode=indexing
          tunnel: [w372] -> w314 mode=indexing
          tunnel: [w371] -> w313 mode=indexing
          tunnel: [w370] -> w312 mode=indexing
          tunnel: [w369] -> w311 mode=indexing
          tunnel: [w368] -> w310 mode=indexing
          tunnel: [w367] -> w309 mode=indexing
          tunnel: [w366] -> w308 mode=indexing
          tunnel: [w365] -> w307 mode=indexing
          n137 = Reshape Array(w364, 9 ("dimension size"), 10 ("dimension size")) -> (w362:dbl[][])
          n138 = Index Array(array=w362, index (col) #1=0, index (col) #2=1, index (col) #3=2, index (col) #4=3, index (col) #5=4, index (col) #6=5, index (col) #7=6, index (col) #8=7, index (col) #9=8) -> (element #1=w361:dbl[], element #2=w360:dbl[], element #3=w359:dbl[], element #4=w358:dbl[], element #5=w357:dbl[], element #6=w356:dbl[], element #7=w355:dbl[], element #8=w354:dbl[], element #9=w353:dbl[])  [unwired: 9 in]
          n139 = Bundle(w374, w361) -> (w373:cluster{dbl[], dbl[]})  [unwired: 1 in]
          n140 = Bundle(w374, w360) -> (w367:cluster{dbl[], dbl[]})  [unwired: 1 in]
          n141 = Bundle(w374, w359) -> (w366:cluster{dbl[], dbl[]})  [unwired: 1 in]
          n142 = Bundle(w374, w358) -> (w365:cluster{dbl[], dbl[]})  [unwired: 1 in]
          n143 = Bundle(w374, w357) -> (w368:cluster{dbl[], dbl[]})  [unwired: 1 in]
          n144 = Bundle(w374, w356) -> (w369:cluster{dbl[], dbl[]})  [unwired: 1 in]
          n145 = Bundle(w374, w355) -> (w370:cluster{dbl[], dbl[]})  [unwired: 1 in]
          n146 = Bundle(w374, w354) -> (w371:cluster{dbl[], dbl[]})  [unwired: 1 in]
          n147 = Bundle(w374, w353) -> (w372:cluster{dbl[], dbl[]})  [unwired: 1 in]
        }
        "Arrhenius 0 V before T change" <- w314
        "Arrhenius 100 V" <- w308
        "Arrhenius - 0 V after T change" <- w315
        "Arrhenius middle 0" <- w310
        "Arrhenius -50 V inc" <- w313
        "Arrhenius -50 V dec" <- w311
        "Arrhenius -100 V" <- w312
        "Arrhenius 50 V dec" <- w307
        "Arrhenius  50 V inc" <- w309
        n148 = call <vilib>:"Add State(s) to Queue__jki_lib_state_machine.vi"("State(s) in (\"\")"=w342) -> ("States Out"=w341:string)  [unwired: 14 in]
      }
      frame "Analysis: Lifespan" {
        w388 = 3600
        # "Template Separator\n(You can make a copy of, or modify, this frame)"
        n149 = Unbundle By Name(w410) -> ("G2T 1D"=w427:cluster{dbl[], dbl[]}[], "G4T 1D"=w426:cluster{dbl[], dbl[]}[], "G2T 2D"=w425:cluster{dbl[], dbl[]}[], "G4T 2D"=w424:cluster{dbl[], dbl[]}[], "Final Temp"=w421:i32, "Init Temp"=w409:i32, "Temp Step"=w408:i32)
        n150 = Subtract(x=w421, y=w409) -> (x-y=w422:i32)
        n151 = Divide(x=w422, y=w408) -> (x/y=w423:dbl)
        n152 = Increment(x=w423) -> (x+1=w407:dbl)
        n153 = for {
          N: w407 -> [_]
          tunnel: w409 -> [w445]
          tunnel: w408 -> [w444]
          tunnel: [w443] -> w406 mode=indexing
          i -> [w446]
          n154 = Multiply(x=w444, y=w446) -> (x*y=w447:i32)
          n155 = Add(x=w445, y=w447) -> (x+y=w443:i32)
        }
        n156 = call <userlib>:"Linear Fit (multiple).vi"("XY-data"=w427) -> ("XY-data out"=w401:cluster{"X-array":dbl[], "Y-array":dbl[]}[], "slopes"=w404:dbl[])  [unwired: 4 in, 5 out]
        n157 = call <userlib>:"Linear Fit (multiple).vi"("XY-data"=w426) -> ("XY-data out"=w400:cluster{"X-array":dbl[], "Y-array":dbl[]}[], "slopes"=w403:dbl[])  [unwired: 4 in, 5 out]
        n158 = call <userlib>:"Linear Fit (multiple).vi"("XY-data"=w425) -> ("XY-data out"=w399:cluster{"X-array":dbl[], "Y-array":dbl[]}[], "slopes"=w402:dbl[])  [unwired: 4 in, 5 out]
        n159 = call <userlib>:"Linear Fit (multiple).vi"("XY-data"=w424) -> ("XY-data out"=w398:cluster{"X-array":dbl[], "Y-array":dbl[]}[], "slopes"=w405:dbl[])  [unwired: 4 in, 5 out]
        n160 = for {
          tunnel: w401 -> [w439] mode=indexing
          tunnel: w400 -> [w440] mode=indexing
          tunnel: w399 -> [w441] mode=indexing
          tunnel: w398 -> [w442] mode=indexing
          tunnel: [w434] -> w397 mode=indexing
          tunnel: [w433] -> w396 mode=indexing
          tunnel: [w432] -> w395 mode=indexing
          tunnel: [w431] -> w394 mode=indexing
          n161 = Unbundle(w439) -> ("Y-array"=w435:dbl[])  [unwired: 1 out]
          n162 = Unbundle(w440) -> ("Y-array"=w436:dbl[])  [unwired: 1 out]
          n163 = Unbundle(w441) -> ("Y-array"=w437:dbl[])  [unwired: 1 out]
          n164 = Unbundle(w442) -> ("Y-array"=w438:dbl[])  [unwired: 1 out]
          n165 = call-poly <vilib>:"Mean.vi"("X"=w438) -> ("mean"=w431:dbl)  [unwired: 1 out]
          n166 = call-poly <vilib>:"Mean.vi"("X"=w437) -> ("mean"=w432:dbl)  [unwired: 1 out]
          n167 = call-poly <vilib>:"Mean.vi"("X"=w436) -> ("mean"=w433:dbl)  [unwired: 1 out]
          n168 = call-poly <vilib>:"Mean.vi"("X"=w435) -> ("mean"=w434:dbl)  [unwired: 1 out]
        }
        n169 = Divide(x=w397, y=w404) -> (x/y=w392:dbl[])
        n170 = Divide(x=w396, y=w403) -> (x/y=w391:dbl[])
        n171 = Divide(x=w395, y=w402) -> (x/y=w390:dbl[])
        n172 = Divide(x=w394, y=w405) -> (x/y=w389:dbl[])
        n173 = Divide(x=w392, y=w388) -> (x/y=w384:dbl[])
        n174 = Divide(x=w391, y=w388) -> (x/y=w385:dbl[])
        n175 = Divide(x=w390, y=w388) -> (x/y=w386:dbl[])
        n176 = Divide(x=w389, y=w388) -> (x/y=w387:dbl[])
        n177 = Array Subset(array=w384, length="Temps to keep (Lifespan)") -> (w415:dbl[])  [unwired: 1 in]
        n178 = Array Subset(array=w385, length="Temps to keep (Lifespan)") -> (w414:dbl[])  [unwired: 1 in]
        n179 = Array Subset(array=w386, length="Temps to keep (Lifespan)") -> (w413:dbl[])  [unwired: 1 in]
        n180 = Array Subset(array=w387, length="Temps to keep (Lifespan)") -> (w412:dbl[])  [unwired: 1 in]
        n181 = Array Subset(array=w406, length="Temps to keep (Lifespan)") -> (w411:i32[])  [unwired: 1 in]
        n182 = Absolute Value(x=w415) -> (abs(x)=w380:dbl[])
        n183 = Absolute Value(x=w414) -> (abs(x)=w381:dbl[])
        n184 = Absolute Value(x=w413) -> (abs(x)=w382:dbl[])
        n185 = Absolute Value(x=w412) -> (abs(x)=w383:dbl[])
        n186 = Bundle(w411, w380) -> (w418:cluster{i32[], dbl[]})  [unwired: 1 in]
        n187 = Bundle(w411, w381) -> (w420:cluster{i32[], dbl[]})  [unwired: 1 in]
        n188 = Bundle(w411, w382) -> (w419:cluster{i32[], dbl[]})  [unwired: 1 in]
        n189 = Bundle(w411, w383) -> (w417:cluster{i32[], dbl[]})  [unwired: 1 in]
        n190 = Build Array(w418, w420, w419, w417) -> (→"Lifespan vs Temp (hrs)":cluster{i32[], dbl[]}[])
        n191 = call <vilib>:"Add State(s) to Queue__jki_lib_state_machine.vi"("State(s) in (\"\")"=w430) -> ("States Out"=w429:string)  [unwired: 14 in]
      }
    }
  }
  "error out" <- w1
